vi "DB_GET PRODUCT TABLE.vi"(11 "PRODUCTS":T1) -> (0 "error out":errorcluster, 1 "Array":string[][](array[string]), 2 "columns":string[](array[string]), 3 "Refnum out":T2)   [LabVIEW 2019, in "CONFIGURATION.lvlib"]
uses:
  Libraries/CONFIGURATION/CONFIGURATION.lvlib
  <vilib>/addons/database/Connection.llb/Conn ObjectReference.ctl
  Libraries/DB_VENDING MACHINE/Type Defs/PRODUCTS.ctl
  <vilib>/addons/database/_DB Variant To Data/Database Variant To Data.xnode
  Libraries/DB_VENDING MACHINE/DB_VENDING MACHINE.lvlib
  <vilib>/addons/database/NI_Database_API.lvlib
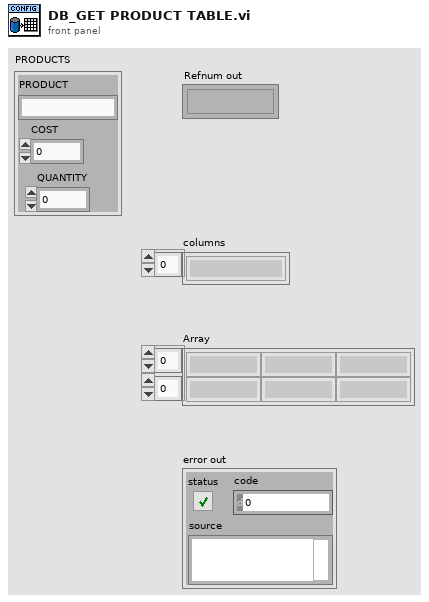
[diagram p1: front panel]
types:
  T1 = typedef "DB_VENDING MACHINE.lvlib/PRODUCTS.ctl" = cluster{"PRODUCT":string, "COST":dbl, "QUANTITY":i8}
  T2 = typedef "NI_Database_API.lvlib/Conn ObjectReference.ctl" = refnum<k1>
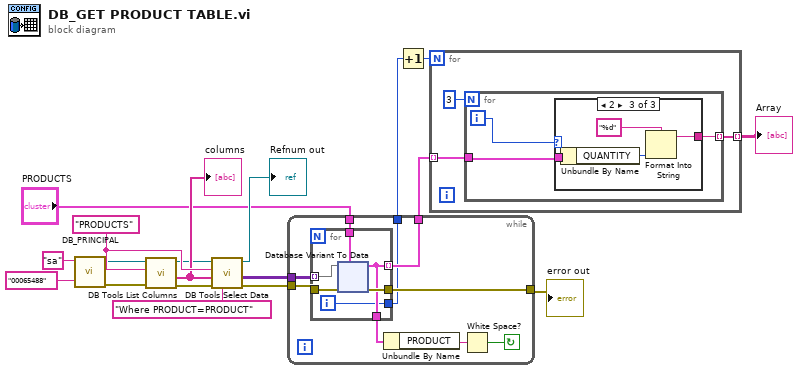
[diagram p0: block diagram]
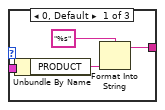
[diagram p2: hidden frame]
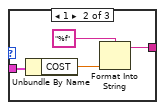
[diagram p3: hidden frame]
diagram:
  w15 = "PRODUCTS" ("table")
  n1 = call "DB_PRINCIPAL.vi"("password"="00065488", "userID"="sa") -> ("error out"=w9:errorcluster, "connection reference"=w8:T2)  [unwired: 8 in]
  n2 = call <vilib>:"DB Tools List Columns.vi"("error in (no error)"=w9, "table"=w15, "connection reference"=w8) -> ("error out"=w13:errorcluster, "columns"=w14:string[], "connection reference out"=w12:T2)  [unwired: 1 in, 1 out]
  "columns" <- w14
  n3 = call <vilib>:"DB Tools Select Data.vi"("condition"="Where PRODUCT=PRODUCT", "error in (no error)"=w13, "columns"=w14, "table"=w15, "connection reference"=w12) -> ("error out"=w6:errorcluster, "data"=w16:variant[][], "connection reference out"=→"Refnum out":T2)  [unwired: 1 in]
  n4 = while {
    tunnel: w16 -> [w27]
    tunnel: w6 -> [w25]
    tunnel: [w24] -> w5
    tunnel: "PRODUCTS" -> [w26]
    tunnel: [w23] -> w4
    tunnel: [w19] -> w3
    stop <- w22 continue-if-true
    n5 = for {
      tunnel: w25 -> [w33]
      tunnel: w26 -> [w32]
      tunnel: w27 -> [w31] mode=indexing
      tunnel: [w29] -> w23 mode=indexing
      tunnel: [w30] -> w24
      tunnel: [w29] -> w20
      tunnel: [w28] -> w19
      i -> [w28]
      n6 = xnode "Database Variant To Data"("database variant"=w31, "error in (no error)"=w33, "type"=w32) -> ("data"=w29:T1, "error out"=w30:errorcluster)
    }
    n7 = Unbundle By Name(w20) -> ("PRODUCT"=w21:string)
    n8 = White Space?(1:w21) -> (0:w22:bool)
  }
  "error out" <- w5
  n9 = Increment(x=w3) -> (x+1=w2:i32)
  n10 = for {
    N: w2 -> [_]
    tunnel: w4 -> [w133] mode=indexing
    tunnel: [w132] -> w7 mode=indexing
    n11 = for {
      N: 3 -> [_]
      tunnel: w133 -> [w136]
      tunnel: [w135] -> w132 mode=indexing
      i -> [w134]
      n12 = case shown="2" w134 {
        tunnel: w136 -> [w140 w144 w148]
        tunnel: [w137 w141 w145] -> w135
        frame 0, Default {
          n13 = Unbundle By Name(w140) -> ("PRODUCT"=w138:string)
          n14 = Format Into String(format string="%s", w138) -> (resulting string=w137:string)  [unwired: 2 in, 1 out]
        }
        frame 1 {
          n15 = Unbundle By Name(w144) -> ("COST"=w142:dbl)
          n16 = Format Into String(format string="%f", w142) -> (resulting string=w141:string)  [unwired: 2 in, 1 out]
        }
        frame 2 {
          n17 = Unbundle By Name(w148) -> ("QUANTITY"=w146:i8)
          n18 = Format Into String(format string="%d", w146) -> (resulting string=w145:string)  [unwired: 2 in, 1 out]
        }
      }
    }
  }
  "Array" <- w7
